vi "ITC503_Split_Cluster.vi"(0 "ITC503-Monitor":T1={"Temperatur (K)"=0.0, "Setpoint (K)"=0.0, "Rate (K/min)"=3.4572, "Heater (%)"=0.0, "NV (%)"=0.0, "Heater Manual"=FALSE, "NV Manual"=FALSE, "Go to Set"=FALSE, "Heater SP"=0.0, "Valid?"=FALSE, "Set Heater SP"=FALSE, "Set NV SP"=FALSE, "Heater (%) Display"=3.4572, "NV (%) Display"=3.4572, "NV Setpoint"=0.0, "Change Heater Status"=FALSE, "Change NV Status"=FALSE, "Sample 3"=0.0, "Sample 2"=0.0, "Sweep-State"=FALSE, "Set Auto PID"=FALSE, "Auto PID"=FALSE, "Stopp"=FALSE, "Setpoint-Sweep"=0.0, "Sample 1"=0.0, "Control Channel"=FALSE, "Channel 1"=FALSE, "Channel 2"=FALSE, "Channel 3"=FALSE} {"NV (%) Display" format="%4_5f"; "Heater (%) Display" format="%4_5f"; "NV (%)" scale=0.0..100.0; "Heater (%)" scale=0.0..100.0; "Rate (K/min)" format="%#4_5f"; "Setpoint (K)" format="%6_5f"}) -> (1 "ITC503-Status-Monitor":T2={"Temperatur (K)"=0.0, "Heater (%)"=0.0, "NV (%)"=0.0, "Heater Manual"=FALSE, "NV Manual"=FALSE, "Valid?"=FALSE, "Heater (%) Display"=3.4572, "NV (%) Display"=3.4572, "Sample 3"=0.0, "Sample 2"=0.0, "Sweep-State"=FALSE, "Auto PID"=FALSE, "Setpoint-Sweep"=0.0, "Sample 1"=0.0, "Channel 1"=FALSE, "Channel 2"=FALSE, "Channel 3"=FALSE} {"NV (%) Display" format="%4_5f"; "Heater (%) Display" format="%4_5f"; "NV (%)" scale=0.0..100.0; "Heater (%)" scale=0.0..100.0}, 2 "ITC503-Control":T3={"Setpoint (K)"=0.0, "Rate (K/min)"=3.4572, "Go to Set"=FALSE, "Set Heater SP"=FALSE, "Set NV SP"=FALSE, "Change Heater Status"=FALSE, "Change NV Status"=FALSE, "Set Auto PID"=FALSE, "Stopp"=FALSE, "Control Channel"=FALSE, "Heater SP"=0.0, "NV Setpoint"=0.0} {"Rate (K/min)" format="%#4_5f"; "Setpoint (K)" format="%6_5f"})   [LabVIEW 2019]
uses:
  ITC503/ITC503_control.ctl
  ITC503/ITC503_Status.ctl
  ITC503/ITC503Monitor-Cluster.ctl
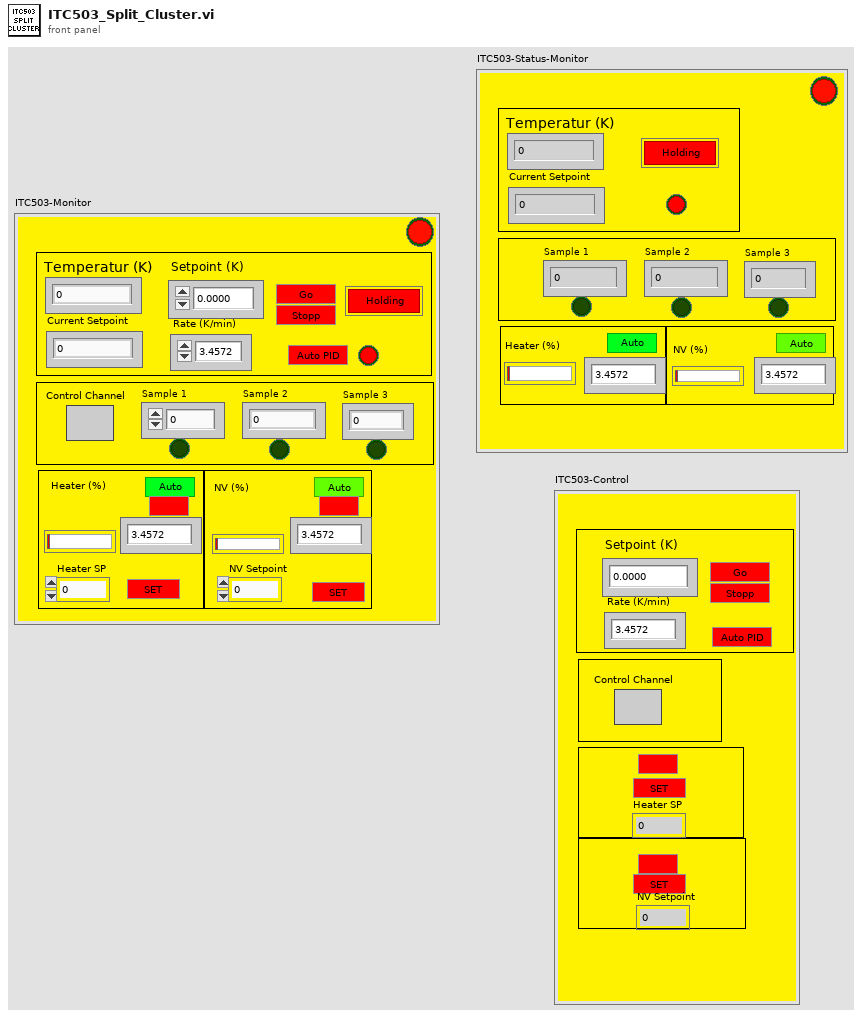
[diagram p1: front panel]
types:
  T1 = typedef "ITC503Monitor-Cluster.ctl" = cluster{"Temperatur (K)":dbl, "Setpoint (K)":dbl, "Rate (K/min)":dbl, "Heater (%)":dbl, "NV (%)":dbl, "Heater Manual":bool, "NV Manual":bool, "Go to Set":bool, "Heater SP":dbl, "Valid?":bool, "Set Heater SP":bool, "Set NV SP":bool, "Heater (%) Display":dbl, "NV (%) Display":dbl, "NV Setpoint":dbl, "Change Heater Status":bool, "Change NV Status":bool, "Sample 3":dbl, "Sample 2":dbl, "Sweep-State":bool, "Set Auto PID":bool, "Auto PID":bool, "Stopp":bool, "Setpoint-Sweep":dbl, "Sample 1":dbl, "Control Channel":bool, "Channel 1":bool, "Channel 2":bool, "Channel 3":bool}
  T2 = typedef "ITC503_Status.ctl" = cluster{"Temperatur (K)":dbl, "Heater (%)":dbl, "NV (%)":dbl, "Heater Manual":bool, "NV Manual":bool, "Valid?":bool, "Heater (%) Display":dbl, "NV (%) Display":dbl, "Sample 3":dbl, "Sample 2":dbl, "Sweep-State":bool, "Auto PID":bool, "Setpoint-Sweep":dbl, "Sample 1":dbl, "Channel 1":bool, "Channel 2":bool, "Channel 3":bool}
  T3 = typedef "ITC503_control.ctl" = cluster{"Setpoint (K)":dbl, "Rate (K/min)":dbl, "Go to Set":bool, "Set Heater SP":bool, "Set NV SP":bool, "Change Heater Status":bool, "Change NV Status":bool, "Set Auto PID":bool, "Stopp":bool, "Control Channel":bool, "Heater SP":dbl, "NV Setpoint":dbl}
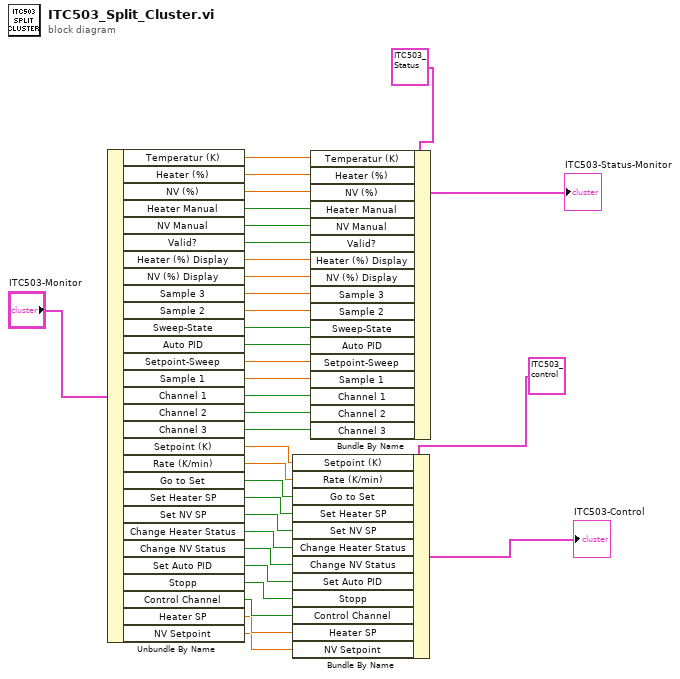
[diagram p0: block diagram]
diagram:
  n1 = Unbundle By Name("ITC503-Monitor") -> ("Temperatur (K)"=w29:dbl, "Heater (%)"=w28:dbl, "NV (%)"=w27:dbl, "Heater Manual"=w26:bool, "NV Manual"=w25:bool, "Valid?"=w24:bool, "Heater (%) Display"=w23:dbl, "NV (%) Display"=w22:dbl, "Sample 3"=w21:dbl, "Sample 2"=w20:dbl, "Sweep-State"=w19:bool, "Auto PID"=w18:bool, "Setpoint-Sweep"=w17:dbl, "Sample 1"=w16:dbl, "Channel 1"=w15:bool, "Channel 2"=w14:bool, "Channel 3"=w13:bool, "Setpoint (K)"=w12:dbl, "Rate (K/min)"=w11:dbl, "Go to Set"=w10:bool, "Set Heater SP"=w9:bool, "Set NV SP"=w8:bool, "Change Heater Status"=w7:bool, "Change NV Status"=w6:bool, "Set Auto PID"=w5:bool, "Stopp"=w4:bool, "Control Channel"=w3:bool, "Heater SP"=w2:dbl, "NV Setpoint"=w1:dbl)
  n2 = Bundle By Name(cluster=T3 {"Setpoint (K)"=0.0, "Rate (K/min)"=3.4572, "Go to Set"=FALSE, "Set Heater SP"=FALSE, "Set NV SP"=FALSE, "Change Heater Status"=FALSE, "Change NV Status"=FALSE, "Set Auto PID"=FALSE, "Stopp"=FALSE, "Control Channel"=FALSE, "Heater SP"=0.0, "NV Setpoint"=0.0} ("ITC503-Control 2"), "Setpoint (K)"=w12, "Rate (K/min)"=w11, "Go to Set"=w10, "Set Heater SP"=w9, "Set NV SP"=w8, "Change Heater Status"=w7, "Change NV Status"=w6, "Set Auto PID"=w5, "Stopp"=w4, "Control Channel"=w3, "Heater SP"=w2, "NV Setpoint"=w1) -> (→"ITC503-Control":T3)
  n3 = Bundle By Name(cluster=T2 {"Temperatur (K)"=0.0, "Heater (%)"=0.0, "NV (%)"=0.0, "Heater Manual"=FALSE, "NV Manual"=FALSE, "Valid?"=FALSE, "Heater (%) Display"=3.4572, "NV (%) Display"=3.4572, "Sample 3"=0.0, "Sample 2"=0.0, "Sweep-State"=FALSE, "Auto PID"=FALSE, "Setpoint-Sweep"=0.0, "Sample 1"=0.0, "Channel 1"=FALSE, "Channel 2"=FALSE, "Channel 3"=FALSE} ("ITC503-Status-Monitor 2"), "Temperatur (K)"=w29, "Heater (%)"=w28, "NV (%)"=w27, "Heater Manual"=w26, "NV Manual"=w25, "Valid?"=w24, "Heater (%) Display"=w23, "NV (%) Display"=w22, "Sample 3"=w21, "Sample 2"=w20, "Sweep-State"=w19, "Auto PID"=w18, "Setpoint-Sweep"=w17, "Sample 1"=w16, "Channel 1"=w15, "Channel 2"=w14, "Channel 3"=w13) -> (→"ITC503-Status-Monitor":T2)
